vi "SetWindowTitle.vi"(8 "No Error":errorcluster, 10 "Title":string, 11 "Window [SDL_Window *]":i64 format="%.0x") -> (0 "Error Out":errorcluster)   [LabVIEW 2026, in "SDL3.lvlib" / "Video.lvlib"]
doc: "<B>Summary</B>\nSet the title of a window."
uses:
  Video.lvlib
  <vilib>/Utility/error.llb/Error Cluster From Error Code.vi
  Error/Error.lvlib
  Lib/SDL3.dll
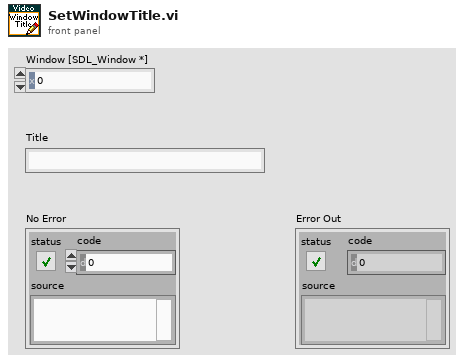
[diagram p1: front panel]
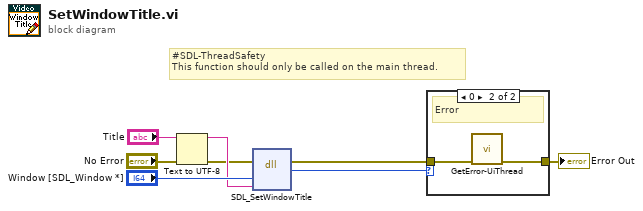
[diagram p0: block diagram]
diagram:
  # "#SDL-ThreadSafety\nThis function should only be called on the main thread."
  n1 = Text to UTF-8(8:"No Error", 11:"Title") -> (0:w1:errorcluster, 3:w2:string)  [unwired: 1 in]
  n2 = dll-call lib="C:/Users/saukko/Dev/LV-SDL3/Sources/SDL3/Lib/SDL3.*" fn="SDL_SetWindowTitle"(error in=w1, "window"="Window [SDL_Window *]", "title"=w2) -> (error out=w6:errorcluster, "return type"=w5:i32)  [unwired: 4 in, 1 out]
  n3 = case shown="0" w5 {
    tunnel: w6 -> [w9 w11]
    tunnel: [w9 w10] -> w8
    frame Default {
      # "Ok"
    }
    frame 0 {
      # "Error"
      n4 = call "GetError-UiThread.vi"("No Error"=w11) -> ("error out"=w10:errorcluster)  [unwired: 10 in]
    }
  }
  "Error Out" <- w8
